vi "Get Cubic Profile State.vi"(8 "Cruise Accel Time":dbl, 9 "Cruise Velocity Time":dbl, 10 "Accel Phases Times":dbl, 11 "Current Time":dbl) -> (3 "Current Stage":T1)   [LabVIEW 2015]
uses:
  Cubic Motion State.ctl
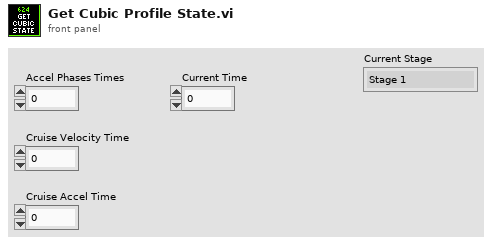
[diagram p1: front panel]
types:
  T1 = typedef "Cubic Motion State.ctl" = enum16{"Stage 1", "Stage 2", "Stage 3", "Stage 4", "Stage 5", "Stage 6", "Stage 7", "Complete"}
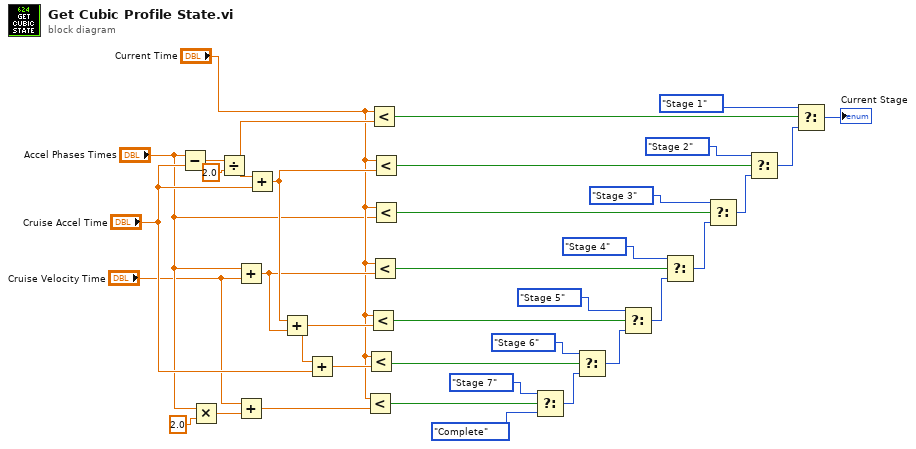
[diagram p0: block diagram]
diagram:
  n1 = Subtract(x="Accel Phases Times", y="Cruise Accel Time") -> (x-y=w33:dbl)
  n2 = Multiply(x="Accel Phases Times", y=2.0) -> (x*y=w3:dbl)
  n3 = Divide(x=w33, y=2.0) -> (x/y=w18:dbl)
  n4 = Add(x="Accel Phases Times", y="Cruise Velocity Time") -> (x+y=w16:dbl)
  n5 = Add(x="Cruise Velocity Time", y=w3) -> (x+y=w1:dbl)
  n6 = Add(x=w18, y="Cruise Accel Time") -> (x+y=w17:dbl)
  n7 = Add(x=w17, y=w16) -> (x+y=w13:dbl)
  n8 = Add(x=w13, y="Cruise Accel Time") -> (x+y=w11:dbl)
  n9 = Less?(x="Current Time", y=w1) -> (x < y?=w7:bool)
  n10 = Less?(x="Current Time", y=w11) -> (x < y?=w14:bool)
  n11 = Less?(x="Current Time", y=w13) -> (x < y?=w23:bool)
  n12 = Less?(x="Current Time", y=w18) -> (x < y?=w35:bool)
  n13 = Less?(x="Current Time", y=w16) -> (x < y?=w26:bool)
  n14 = Less?(x="Current Time", y=w17) -> (x < y?=w30:bool)
  n15 = Less?(x="Current Time", y="Accel Phases Times") -> (x < y?=w29:bool)
  n16 = Select(t=Cubic_Motion_State."Stage 7", s=w7, f=Cubic_Motion_State."Complete") -> (s? t:f=w8:T1)
  n17 = Select(t=Cubic_Motion_State."Stage 6", s=w14, f=w8) -> (s? t:f=w15:T1)
  n18 = Select(t=Cubic_Motion_State."Stage 5", s=w23, f=w15) -> (s? t:f=w21:T1)
  n19 = Select(t=Cubic_Motion_State."Stage 4", s=w26, f=w21) -> (s? t:f=w24:T1)
  n20 = Select(t=Cubic_Motion_State."Stage 3", s=w29, f=w24) -> (s? t:f=w27:T1)
  n21 = Select(t=Cubic_Motion_State."Stage 2", s=w30, f=w27) -> (s? t:f=w31:T1)
  n22 = Select(t=Cubic_Motion_State."Stage 1", s=w35, f=w31) -> (s? t:f=→"Current Stage":T1)
